vi "New Report.vi"(8 "error in (no error)":errorcluster) -> (0 "error out":errorcluster)   [LabVIEW 2020, in "Astemes_CSVReportPlugin.lvlib" / "Report Generator.lvlib"]
uses:
  Report Generator.lvlib
  Private/Reference.vi
  Test Result Handler/TestStand Result Handler.lvclass
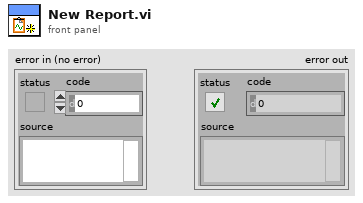
[diagram p1: front panel]
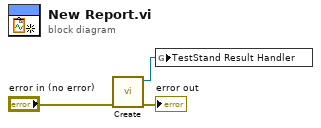
[diagram p0: block diagram]
diagram:
  n1 = call "Create.vi"("error in (no error)"="error in (no error)") -> ("error out"=→"error out":errorcluster, "Test Result Handler"=w3:refnum<class "TestStand Result Handler.lvclass">)  [unwired: 9 in]
  n2 = global write "Reference.vi" "TestStand Result Handler"(w3) -> ()
